vi "CHS_TRAJECTORY_DASH_WRITE.vi"   [LabVIEW 2019]
uses:
  CHS_TRAJECTORY_GLOBALS.vi
  <vilib>/Rock Robotics/Network Tables/NT Write Number.vi
  <vilib>/Rock Robotics/Network Tables/NT Write Boolean.vi
  <vilib>/Rock Robotics/Network Tables/NT Write Numeric Array.vi
types:
  T1 = typedef "Trajectory_Library.lvlib/POSE2D.ctl" = cluster{"TRANSLATION":T2, "ROTATION":T3}
  T2 = typedef "Trajectory_Library.lvlib/TRANSLATION2D.ctl" = cluster{"X":dbl, "Y":dbl}
  T3 = typedef "Trajectory_Library.lvlib/ROTATION2D.ctl" = cluster{"VALUE":dbl, "COS":dbl, "SIN":dbl}
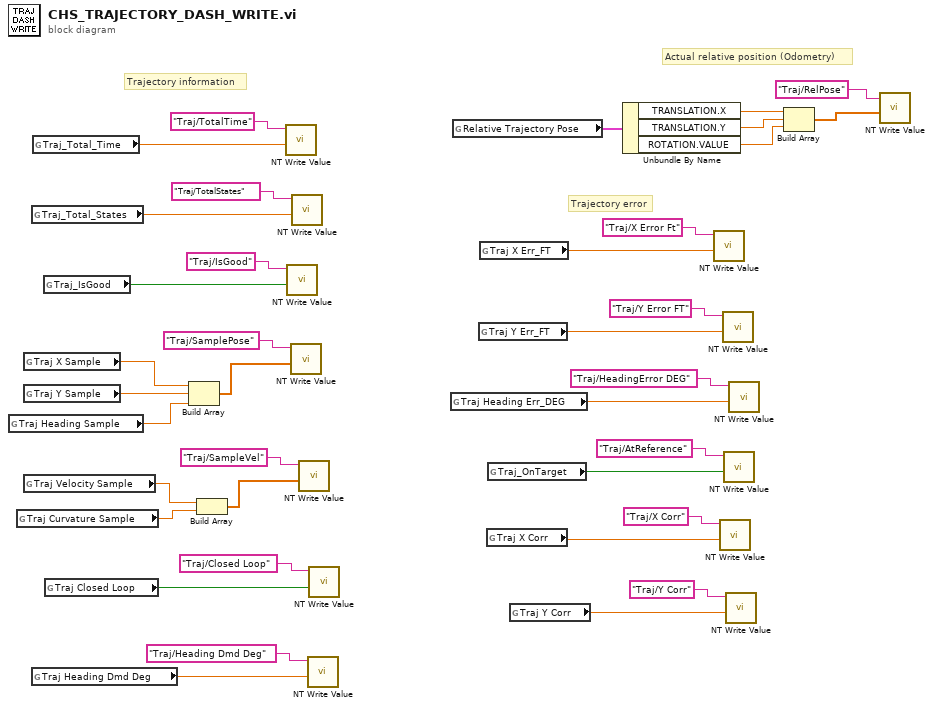
[diagram p0: block diagram]
diagram:
  # "Trajectory information"
  # "Actual relative position (Odometry)"
  # "Trajectory error"
  n1 = global read "CHS_TRAJECTORY_GLOBALS.vi" "Traj Heading Sample"() -> (w12:dbl)
  n2 = global read "CHS_TRAJECTORY_GLOBALS.vi" "Traj Curvature Sample"() -> (w10:dbl)
  n3 = global read "CHS_TRAJECTORY_GLOBALS.vi" "Traj X Sample"() -> (w14:dbl)
  n4 = global read "CHS_TRAJECTORY_GLOBALS.vi" "Traj Y Sample"() -> (w13:dbl)
  n5 = global read "CHS_TRAJECTORY_GLOBALS.vi" "Traj Velocity Sample"() -> (w11:dbl)
  n6 = global read "CHS_TRAJECTORY_GLOBALS.vi" "Traj_Total_States"() -> (w16:dbl)
  n7 = global read "CHS_TRAJECTORY_GLOBALS.vi" "Traj Heading Dmd Deg"() -> (w8:dbl)
  n8 = global read "CHS_TRAJECTORY_GLOBALS.vi" "Traj_Total_Time"() -> (w15:dbl)
  n9 = global read "CHS_TRAJECTORY_GLOBALS.vi" "Traj_IsGood"() -> (w17:bool)
  n10 = global read "CHS_TRAJECTORY_GLOBALS.vi" "Traj Closed Loop"() -> (w9:bool)
  n11 = Build Array(w14, w13, w12) -> (w31:dbl[])
  n12 = Build Array(w11, w10) -> (w33:dbl[])
  n13 = call-poly <vilib>:"NT Write Value.vi"("Numeric"=w15, "Name"="Traj/TotalTime") -> ()  [unwired: 9 in, 1 out]
  n14 = call-poly <vilib>:"NT Write Value.vi"("Boolean"=w17, "Name"="Traj/IsGood") -> ()  [unwired: 9 in, 1 out]
  n15 = call-poly <vilib>:"NT Write Value.vi"("Numeric Array"=w31, "Name"="Traj/SamplePose") -> ()  [unwired: 9 in, 1 out]
  n16 = call-poly <vilib>:"NT Write Value.vi"("Numeric"=w16, "Name"="Traj/TotalStates") -> ()  [unwired: 9 in, 1 out]
  n17 = call-poly <vilib>:"NT Write Value.vi"("Numeric Array"=w33, "Name"="Traj/SampleVel") -> ()  [unwired: 9 in, 1 out]
  n18 = call-poly <vilib>:"NT Write Value.vi"("Numeric"=w8, "Name"="Traj/Heading Dmd Deg") -> ()  [unwired: 9 in, 1 out]
  n19 = call-poly <vilib>:"NT Write Value.vi"("Boolean"=w9, "Name"="Traj/Closed Loop") -> ()  [unwired: 9 in, 1 out]
  n20 = global read "CHS_TRAJECTORY_GLOBALS.vi" "Traj Heading Err_DEG"() -> (w5:dbl)
  n21 = global read "CHS_TRAJECTORY_GLOBALS.vi" "Relative Trajectory Pose"() -> (w1:T1)
  n22 = global read "CHS_TRAJECTORY_GLOBALS.vi" "Traj Y Err_FT"() -> (w7:dbl)
  n23 = global read "CHS_TRAJECTORY_GLOBALS.vi" "Traj X Err_FT"() -> (w6:dbl)
  n24 = global read "CHS_TRAJECTORY_GLOBALS.vi" "Traj X Corr"() -> (w2:dbl)
  n25 = global read "CHS_TRAJECTORY_GLOBALS.vi" "Traj_OnTarget"() -> (w4:bool)
  n26 = global read "CHS_TRAJECTORY_GLOBALS.vi" "Traj Y Corr"() -> (w3:dbl)
  n27 = Unbundle By Name(w1) -> ("TRANSLATION.X"=w27:dbl, "TRANSLATION.Y"=w28:dbl, "ROTATION.VALUE"=w29:dbl)
  n28 = call-poly <vilib>:"NT Write Value.vi"("Numeric"=w6, "Name"="Traj/X Error Ft") -> ()  [unwired: 9 in, 1 out]
  n29 = call-poly <vilib>:"NT Write Value.vi"("Numeric"=w2, "Name"="Traj/X Corr") -> ()  [unwired: 9 in, 1 out]
  n30 = call-poly <vilib>:"NT Write Value.vi"("Numeric"=w7, "Name"="Traj/Y Error FT") -> ()  [unwired: 9 in, 1 out]
  n31 = call-poly <vilib>:"NT Write Value.vi"("Boolean"=w4, "Name"="Traj/AtReference") -> ()  [unwired: 9 in, 1 out]
  n32 = call-poly <vilib>:"NT Write Value.vi"("Numeric"=w3, "Name"="Traj/Y Corr") -> ()  [unwired: 9 in, 1 out]
  n33 = call-poly <vilib>:"NT Write Value.vi"("Numeric"=w5, "Name"="Traj/HeadingError DEG") -> ()  [unwired: 9 in, 1 out]
  n34 = Build Array(w27, w28, w29) -> (w25:dbl[])
  n35 = call-poly <vilib>:"NT Write Value.vi"("Numeric Array"=w25, "Name"="Traj/RelPose") -> ()  [unwired: 9 in, 1 out]
